vi "Table_ScrollaBarMarvin.vi"(3 "error in":errorcluster, 4 "Line to focus":string, 5 "reference in":refnum<vi>) -> (0 "error out":errorcluster, 1 "OK?":bool, 2 "reference out":refnum<vi>)   [LabVIEW 2017]
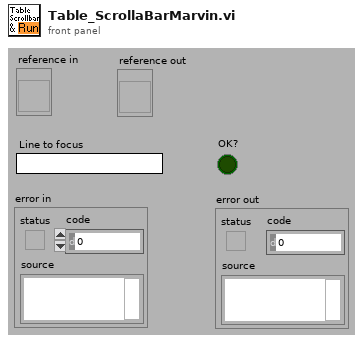
[diagram p1: front panel]
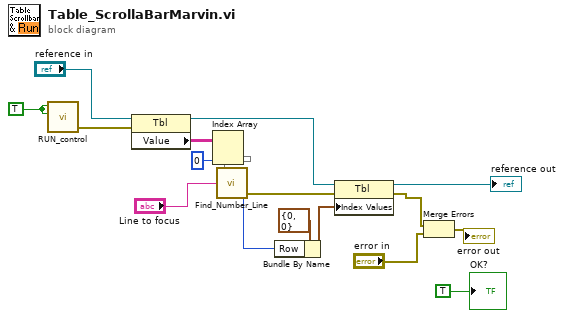
[diagram p0: block diagram]
diagram:
  w4 = TRUE ("Blinking")
  n1 = call "RUN_control.vi"("Blinking(:T)"=w4, "Value (:T)"=w4) -> ("error out"=w5:errorcluster)  [unwired: 3 in, 2 out]
  n2 = property on="Property Node" class="Tbl"(reference="reference in", error in=w5) -> (reference out=w6:refnum<vi>, "Value"=w2:string[][])  [unwired: 1 out]
  n3 = Index Array(array=w2, index (col)=0 ("disabled index (col)")) -> (element=w1:string[])  [unwired: 1 in]
  n4 = call "Find_Number_Line.vi"("Test Paragraph"="Line to focus", "Row Headers[]"=w1) -> ("error out"=w13:errorcluster, "Line number"=w15:i32)  [unwired: 1 in, 1 out]
  n5 = Bundle By Name(cluster=cluster{"Row":i32, "Column":i32} {"Row"=0, "Column"=0} ("Edit Position"), "Row"=w15) -> (w16:cluster{"Row":i32, "Column":i32})
  n6 = property on="Property Node" class="Tbl"(reference=w6, error in=w13, "Index Values"=w16) -> (reference out=→"reference out":refnum<vi>, error out=w9:errorcluster)
  n7 = Merge Errors(w9, "error in") -> (→"error out":errorcluster)
  "OK?" <- TRUE ("OK?")
